vi "Read VI Server Configuration.vi"(8 "error in (no error)":errorcluster, 11 "VI Server Recorder in":refnum<class "VI Server Recorder.lvclass">) -> (0 "error out":errorcluster, 2 "VI Server Configuration":T1, 3 "VI Server Recorder out":refnum<class "VI Server Recorder.lvclass">)   [LabVIEW 2019, in "VI Server Recorder.lvclass"]
uses:
  VI Server Recorder.lvclass
  C:/GitHub/LabActor/Template Module/Template Module.lvclass
  VI Server Configuration.ctl
  Template Module/Template Module.lvclass/Template Module.ctl
  Template Module/Read Configuration.vi
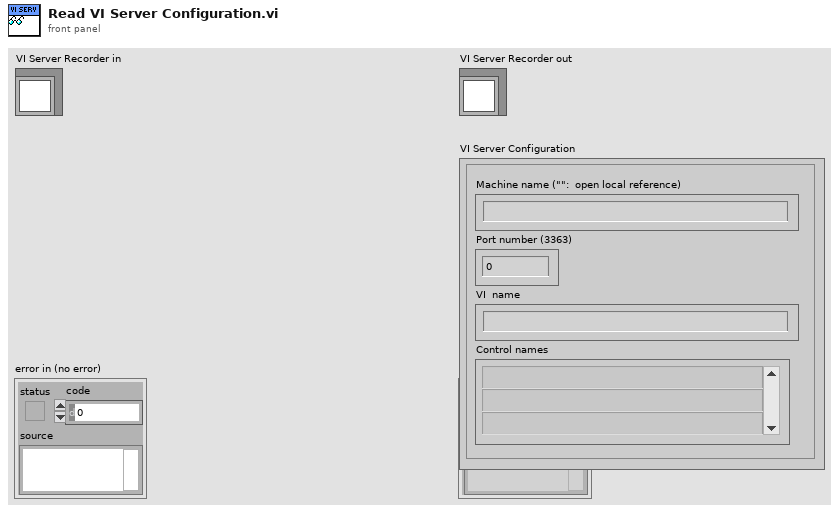
[diagram p1: front panel]
types:
  T1 = typedef "VI Server Configuration.ctl" = cluster{"Machine name (\"\":  open local reference)":string, "Port number (3363)":u16, "Control names":string[], "VI  name":string}
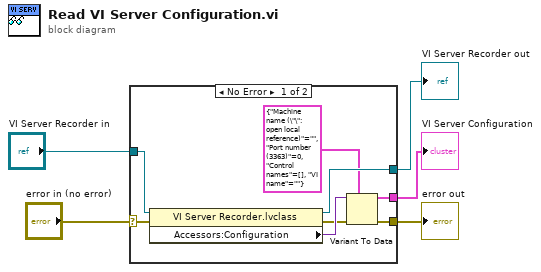
[diagram p0: block diagram]
diagram:
  n1 = case shown="No Error" "error in (no error)" {
    selector: "error in (no error)" -> [w13 w14]
    tunnel: [w7 w14] -> w4
    tunnel: [w11 w15] -> w2
    tunnel: "VI Server Recorder in" -> [w12 w15]
    tunnel: [w8 _] -> w1
    frame No Error {
      n2 = property class="VI Server Recorder.lvclass"(reference=w12, error in=w13) -> (reference out=w11:refnum<class "VI Server Recorder.lvclass">, error out=w6:errorcluster, "Accessors:Configuration"=w10:variant)
      n3 = Variant To Data(error in=w6, type=T1 {"Machine name (\"\":  open local reference)"="", "Port number (3363)"=0, "Control names"=[], "VI  name"=""} ("VI Server Configuration"), Variant=w10) -> (data=w8:T1, error out=w7:errorcluster)
    }
    frame Error {
    }
  }
  "error out" <- w4
  "VI Server Recorder out" <- w2
  "VI Server Configuration" <- w1
